vi "Set Message Stream.vi"(10 "Message Stream.lvclass":refnum<class "Message Stream.lvclass">, 11 "CRIO MSS Test Actor in":refnum<class "MSS Target Actor.lvclass">) -> (3 "CRIO MSS Test Actor out":refnum<class "MSS Target Actor.lvclass">)   [LabVIEW 2024, in "MSS Target Actor.lvlib" / "MSS Target Actor.lvclass"]
uses:
  MSS Target Actor.lvclass
  <vilib>/ni/Actors/Network Endpoint Actors/Abstract Classes/Message Stream/Message Stream.lvclass
  MSS Target Actor.lvclass/MSS Target Actor.ctl
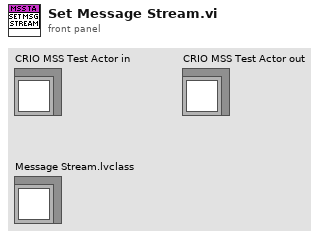
[diagram p1: front panel]
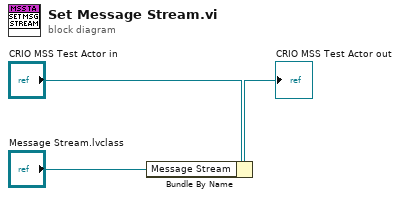
[diagram p0: block diagram]
diagram:
  n1 = Bundle By Name(cluster="CRIO MSS Test Actor in", "Message Stream"="Message Stream.lvclass") -> (→"CRIO MSS Test Actor out":refnum<class "MSS Target Actor.lvclass">)
